vi "Move_Until_Position.vi"(8 "error in (no error)":errorcluster, 9 "Z-Position":dbl=50.0 format="%#_13g", 10 "index":i32, 11 "VISA Refnum in":refnum<visa-resource-name>) -> (0 "error out":errorcluster, 3 "VISA Refnum out":refnum<visa-resource-name>)   [LabVIEW 2018]
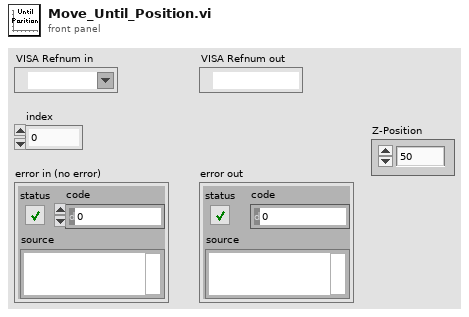
[diagram p1: front panel]
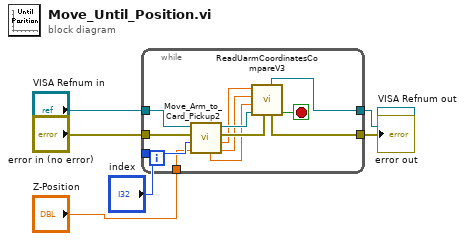
[diagram p0: block diagram]
diagram:
  n1 = while {
    tunnel: "index" -> [w16]
    tunnel: "Z-Position" -> [w7]
    tunnel: "VISA Refnum in" -> [w18]
    tunnel: [w13] -> w5
    tunnel: "error in (no error)" -> [w17]
    tunnel: [w12] -> w6
    stop <- w8 stop-if-true
    n2 = call "Move_Arm_to_Card_Pickup2.vi"("Z-Position"=w7, "index"=w16, "error in"=w17, "Machine In"=w18) -> ("X Coordinate"=w10:dbl, "Y Coordinate"=w11:dbl, "error out"=w15:errorcluster, "Machine Out"=w14:refnum<visa-resource-name>, "Z Coordinate"=w9:dbl)  [unwired: 3 in]
    n3 = call "ReadUarmCoordinatesCompareV3.vi"("error in"=w15, "Machine In"=w14, "INPUT Z Coord"=w9, "INPUT X Coord"=w10, "INPUT Y Coord"=w11) -> ("x = y?"=w8:bool, "error out"=w12:errorcluster, "Machine Out"=w13:refnum<visa-resource-name>)  [unwired: 1 in, 3 out]
  }
  "error out" <- w6
  "VISA Refnum out" <- w5
